vi "Replace Formatting with Tags.vi"(7 "Set Value? (T)":bool, 8 "error in (no error)":errorcluster, 9 "Length":i32[](array[numeric]), 10 "Start":i32[](array[numeric]), 11 "String Ref":refnum<vi>) -> (0 "error out":errorcluster, 2 "New String":string, 3 "String Ref out":refnum<vi>)   [LabVIEW 2020, in "VI Properties Editor.lvlib"]
doc: "Replaces bold formatting with bold tags in the locations specified."
uses:
  VI Properties Editor.lvlib
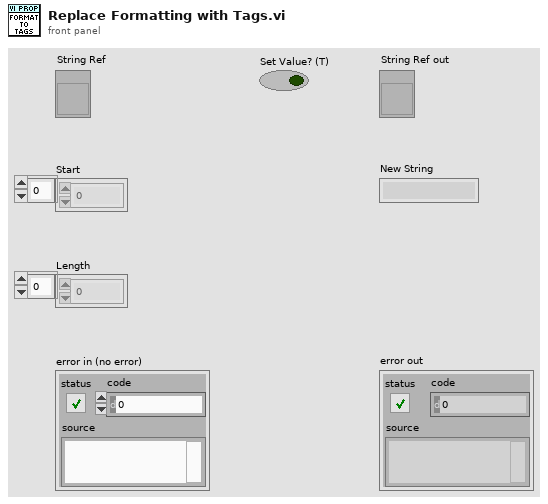
[diagram p1: front panel]
types:
  T1 = typedef "LVSelectionTypeDef.ctl" = cluster{"Selection Start":u32, "Selection End":u32}
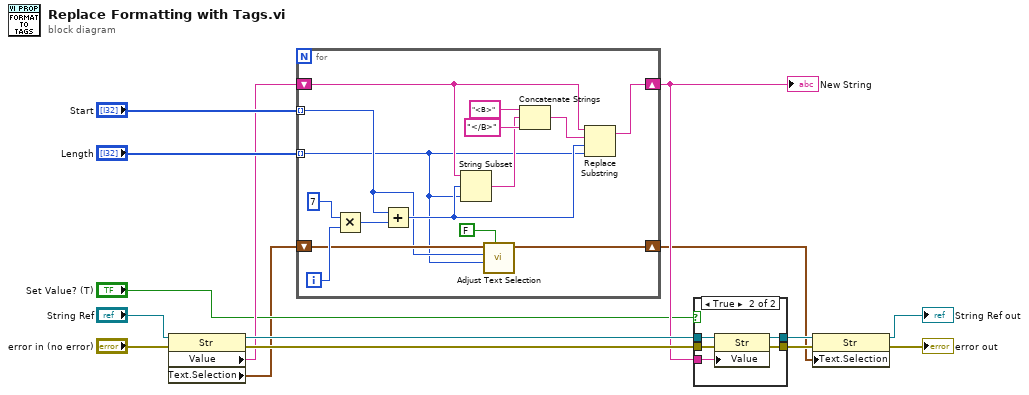
[diagram p0: block diagram]
diagram:
  n1 = property class="Str"(reference="String Ref", error in="error in (no error)") -> (reference out=w10:refnum<vi>, error out=w11:errorcluster, "Value"=w8:string, "Text.Selection"=w2:T1)
  n2 = for {
    tunnel: "Length" -> [w18] mode=indexing
    tunnel: "Start" -> [w19] mode=indexing
    shift-right: [w27] -> w9
    shift-left: w8 -> [w22]
    shift-right: [w17] -> w1
    shift-left: w2 -> [w20]
    i -> [w25]
    n3 = Multiply(x=7, y=w25) -> (x*y=w23:i32)
    n4 = Add(x=w19, y=w23) -> (x+y=w21:i32)
    n5 = String Subset(string=w22, offset (0)=w21, length (rest)=w18) -> (substring=w28:string)
    n6 = call "Adjust Text Selection.vi"("Remove?"=FALSE, "Length"=w18, "Start"=w19, "Selection"=w20) -> ("Selection out"=w17:T1)  [unwired: 7 in]
    n7 = Concatenate Strings("<B>" ("string"), w28, "</B>" ("string")) -> (w26:string)
    n8 = Replace Substring(2:w18, 3:w21, 4:w26, 5:w22) -> (1:w27:string)  [unwired: 1 out]
  }
  "New String" <- w9
  n9 = case shown="True" "Set Value? (T)" {
    tunnel: w11 -> [w32 w37]
    tunnel: [w32 w36] -> w5
    tunnel: w10 -> [w31 w35]
    tunnel: [w31 w34] -> w6
    tunnel: w9 -> [_ w33]
    frame False {
    }
    frame True {
      n10 = property class="Str"(reference=w35, error in=w37, "Value"=w33) -> (reference out=w34:refnum<vi>, error out=w36:errorcluster)
    }
  }
  n11 = property class="Str"(reference=w6, error in=w5, "Text.Selection"=w1) -> (reference out=→"String Ref out":refnum<vi>, error out=→"error out":errorcluster)
